vi "Write Position_Tiles.vi"(8 "error in (no error)":errorcluster, 10 "Coordinate":T1, 11 "BounceTarget in":refnum<class "BounceTarget.lvclass">) -> (0 "error out":errorcluster, 3 "BounceTarget out":refnum<class "BounceTarget.lvclass">)   [LabVIEW 2019, in "RT_Game.lvlib" / "BounceTarget.lvclass"]
uses:
  BounceTarget.lvclass
  C:/Users/FreshBob/Dropbox/VIs/myRIO_GameConsole/RT/RT_Game/GameObject/GameObject.lvclass
  Game/Coordinate.ctl
  GameObject/GameObject.lvclass/GameObject.ctl
  BounceTarget.lvclass/BounceTarget.ctl
  GameObject/Write position.vi
  Game/Game.lvclass
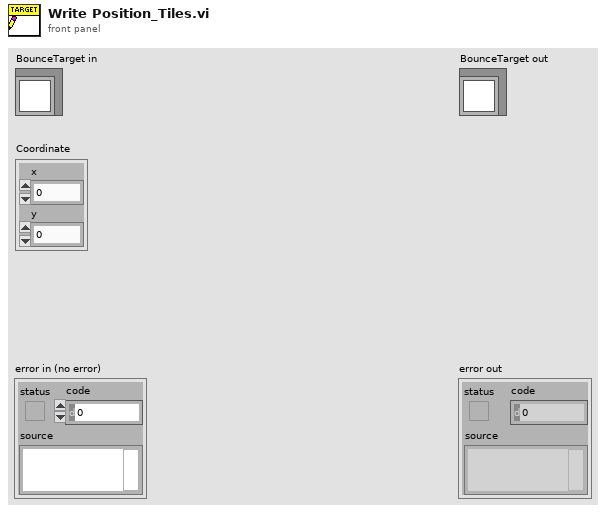
[diagram p1: front panel]
types:
  T1 = typedef "RT_Game.lvlib/Game.lvclass/Coordinate.ctl" = cluster{"x":dbl, "y":dbl}
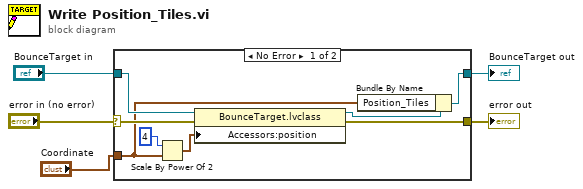
[diagram p0: block diagram]
diagram:
  n1 = case shown="No Error" "error in (no error)" {
    selector: "error in (no error)" -> [w13 w14]
    tunnel: [w11 w14] -> w4
    tunnel: [w12 w15] -> w2
    tunnel: "BounceTarget in" -> [w10 w15]
    tunnel: "Coordinate" -> [w8 _]
    frame No Error {
      n2 = Scale By Power Of 2(n=i16 4, x=w8) -> (x*2^n=w7:T1)
      n3 = property class="BounceTarget.lvclass"(reference=w10, error in=w13, "Accessors:position"=w7) -> (reference out=w9:refnum<class "BounceTarget.lvclass">, error out=w11:errorcluster)
      n4 = Bundle By Name(cluster=w9, "Position_Tiles"=w8) -> (w12:refnum<class "BounceTarget.lvclass">)
    }
    frame Error {
    }
  }
  "error out" <- w4
  "BounceTarget out" <- w2
